vi "Process Job.vi"(8 "error in (no error)":errorcluster, 10 "Task":refnum<class>, 11 "Barista in":refnum<class "Barista.lvclass">) -> (0 "error out":errorcluster, 3 "Barista out":refnum<class "Barista.lvclass">)   [LabVIEW 2023, in "Barista.lvclass"]
doc: "Perform the task assigned by the work dispatcher. This VI is an override of a generic method all descendants of the Worker class must implement. \n\nThis method, being implemented by the Barista class, handles the actual making of drinks in the coffee shop."
uses:
  Barista.lvclass
  Order/Order Item.lvclass
  Worker.lvclass
panel:
  in  "Customer Left":string="Customer left before their drink was ready!\nItem: %s\nThe staff enjoyed drinking it instead."
  in  "Making Drink":string="Making drink for %s"
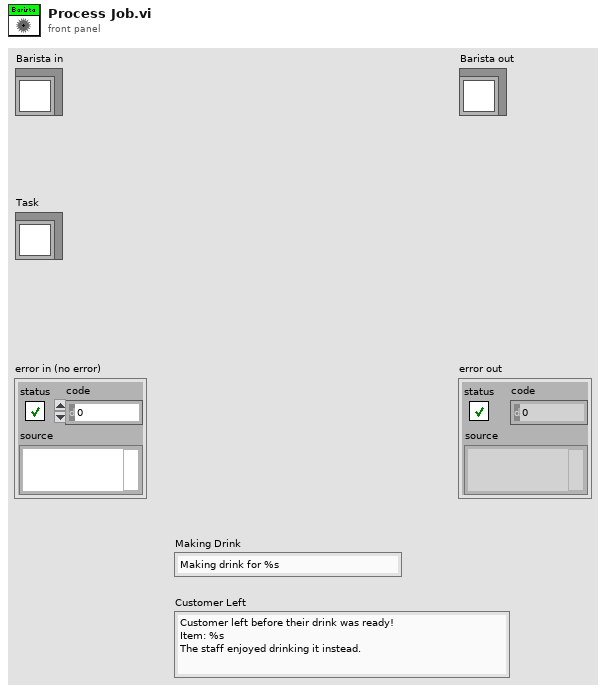
[diagram p1: front panel]
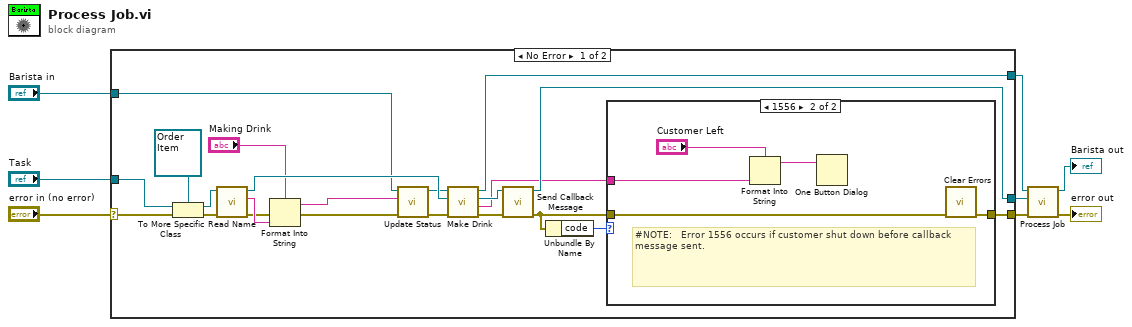
[diagram p0: block diagram]
diagram:
  n1 = case shown="No Error" "error in (no error)" {
    selector: "error in (no error)" -> [w14 w39]
    tunnel: [w22 w39] -> w1
    tunnel: "Barista in" -> [w11 w38]
    tunnel: [w27 w38] -> w5
    tunnel: "Task" -> [w30 w37]
    tunnel: [w28 w37] -> w2
    frame No Error {
      n2 = To More Specific Class(target class=refnum<class "Order Item.lvclass"> refnum ("Order Item.lvclass"), reference=w30, error in=w14) -> (specific class reference=w19:refnum<class "Order Item.lvclass">, error out=w20:errorcluster)
      n3 = call-dynamic "Read Name.vi"("error in (no error)"=w20, "Order Item in"=w19) -> ("error out"=w15:errorcluster, "Name"=w16:string, "Order Item out"=w18:refnum<class "Order Item.lvclass">)  [unwired: 7 in]
      n4 = Format Into String(format string="Making Drink", error in=w15, w16) -> (resulting string=w13:string, error out=w12:errorcluster)  [unwired: 1 in]
      n5 = call-dynamic "Update Status.vi"("error in (no error)"=w12, "Status"=w13, "Worker in"=w11) -> ("error out"=w9:errorcluster, "Worker out"=w10:refnum<class "Barista.lvclass">)  [unwired: 7 in]
      n6 = call-dynamic "Make Drink.vi"("error in (no error)"=w9, "Order Item in"=w18, "Barista in"=w10) -> ("error out"=w26:errorcluster, "Description"=w21:string, "Order Item out"=w25:refnum<class "Order Item.lvclass">, "Barista out"=w27:refnum<class "Barista.lvclass">)  [unwired: 5 in]
      n7 = call-dynamic "Send Callback Message.vi"("error in (no error)"=w26, "Order Item in"=w25) -> ("error out"=w23:errorcluster, "Order Item out"=w28:refnum<class "Order Item.lvclass">)  [unwired: 8 in]
      n8 = Unbundle By Name(w23) -> ("code"=w24:i32)
      n9 = case shown="1556" w24 {
        tunnel: w23 -> [w31 w36]
        tunnel: [w31 w35] -> w22
        tunnel: w21 -> [_ w32]
        frame Default {
        }
        frame 1556 {
          # "#NOTE:   Error 1556 occurs if customer shut down before callback message sent."
          n10 = Format Into String(format string="Customer Left", w32) -> (resulting string=w34:string)  [unwired: 2 in, 1 out]
          n11 = One Button Dialog(message=w34) -> ()  [unwired: 1 in, 1 out]
          n12 = call <vilib>:"Clear Errors.vi"("error in (no error)"=w36) -> ("error out"=w35:errorcluster)  [unwired: 5 in, 1 out]
        }
      }
    }
    frame Error {
    }
  }
  n13 = call-parent "Process Job.vi"("error in"=w1, "Task"=w2, "Worker in"=w5) -> ("error out"=→"error out":errorcluster, "Worker out"=→"Barista out":refnum<class "Barista.lvclass">)  [unwired: 7 in]
